vi "DAQmx Create Channel (TEDS-AI-Force-IEPE Sensor).vi"(0 "task in":refnum<k21>, 1 "maximum value":dbl=2000.0 format="%0.2f", 2 "minimum value":dbl=-2000.0 format="%0.2f", 3 "input terminal configuration":i32(ring)=-1 items=["default"=-1, "RSE"=10083, "NRSE"=10078, "Differential"=10106, "Pseudodifferential"=12529], 5 "physical channels":tag, 6 "current excitation source":i32(ring)=10200 items=["Internal"=10200, "External"=10167, "None"=10230], 7 "name to assign":string, 8 "current excitation value":dbl=0.001, 9 "units":i32(ring)=15875 items=["Newtons"=15875, "Pounds"=15876, "kgf"=15877, "From Custom Scale"=10065], 11 "error in":errorcluster, 12 "custom scale name":tag) -> (4 "task out":refnum<k21>, 15 "error out":errorcluster)   [LabVIEW 2011]
doc: "Creates channel(s) that use an IEPE force sensor to measure force or load. You must configure the physical channel(s) with TEDS information to use this VI."
uses:
  C:/Program Files/National Instruments/LabVIEW 2011/resource/objmgr/daqmx.rc
panel:
  # "input limits"
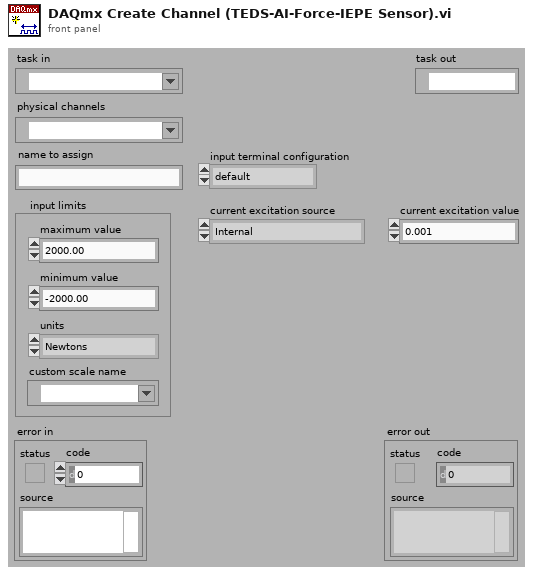
[diagram p1: front panel]
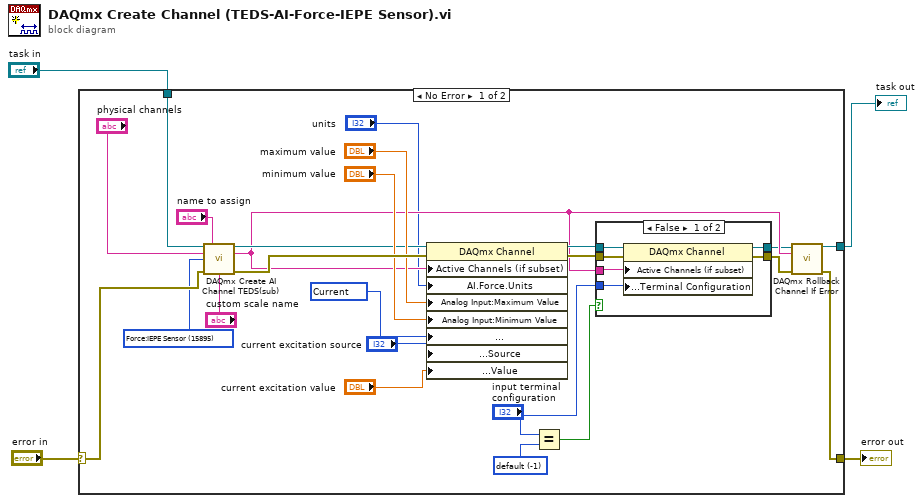
[diagram p0: block diagram]
diagram:
  n1 = case shown="No Error" "error in" {
    selector: "error in" -> [w27 w38]
    tunnel: [w18 w38] -> w2
    tunnel: "task in" -> [w28 w37]
    tunnel: [w19 w37] -> w1
    frame No Error {
      w5 = 15895 items=["Voltage"=10322, "Current"=10134, "More:Voltage:Custom with Excitation"=10323, "More:Current:Custom with Excitation"=10136, "Frequency"=10181, "Period"=10257, "Resistance"=10278, "Temperature:Thermocouple"=10303, "Temperature:Thermistor"=10302, "Temperature:RTD"=10301, "Temperature:Built-in Sensor"=10311, "Strain Gage"=10300, "LVDT"=10352, "RVDT"=10353, "Accelerometer:Voltage Input"=10355, "Accelerometer:Current Input"=10356, "Force:IEPE Sensor"=15895] ("measurement type")
      w9 = -1 items=["default"=-1, "differential"=10106, "RSE"=10083, "NRSE"=10078] ("input terminal configuration")
      w15 = 10134 items=["Voltage"=10322, "Current"=10134] ("AI.Excit.VoltageOrCurrent")
      n2 = call "DAQmx Create AI Channel TEDS(sub).vi"("task in"=w28, "virtual channel name"="name to assign", "physical channel name"="physical channels", "measurement type"=w5, "error in"=w27, "custom scale"="custom scale name") -> ("task out"=w20:refnum<k21>, "channel names"=w12:string, "error out"=w24:errorcluster)  [unwired: 7 out]
      n3 = property class="DAQmx Channel"(reference=w20, error in=w24, "Active Channels (if subset)"=w12, "AI.Force.Units"="units", "Analog Input:Maximum Value"="maximum value", "Analog Input:Minimum Value"="minimum value", "Analog Input:General Properties:Signal Conditioning:Excitation:Advanced:Voltage or Current"=w15, "Analog Input:General Properties:Signal Conditioning:Excitation:Source"="current excitation source", "Analog Input:General Properties:Signal Conditioning:Excitation:Value"="current excitation value") -> (reference out=w14:refnum<k21>, error out=w13:errorcluster)
      n4 = Equal?(x="input terminal configuration", y=w9) -> (x = y?=w7:bool)
      n5 = case shown="False" w7 {
        tunnel: w13 -> [w34 w36]
        tunnel: [w33 w35] -> w11
        tunnel: [w32 w36] -> w10
        tunnel: "input terminal configuration" -> [w31 _]
        tunnel: w12 -> [w30 _]
        tunnel: w14 -> [w29 w35]
        frame False {
          n6 = property class="DAQmx Channel"(reference=w29, error in=w34, "Active Channels (if subset)"=w30, "Analog Input:General Properties:Input Configuration:Terminal Configuration"=w31) -> (reference out=w33:refnum<k21>, error out=w32:errorcluster)
        }
        frame True {
        }
      }
      n7 = call "DAQmx Rollback Channel If Error.vi"("task in"=w11, "channel names"=w12, "error in"=w10) -> ("task out"=w19:refnum<k21>, "error out"=w18:errorcluster)  [unwired: 11 out]
    }
    frame Error {
    }
  }
  "error out" <- w2
  "task out" <- w1
